vi "DO State Machine (array).vi"(0 "FPGA DO Loop Data in":T1={"DO"=[FALSE, FALSE, FALSE, FALSE, FALSE, FALSE, FALSE, FALSE, FALSE, FALSE, FALSE, FALSE, FALSE, FALSE, FALSE, FALSE, FALSE, FALSE, FALSE, FALSE, FALSE, FALSE, FALSE, FALSE, FALSE, FALSE, FALSE, FALSE, FALSE, FALSE, FALSE, FALSE], "Is Pulse"=[FALSE, FALSE, FALSE, FALSE, FALSE, FALSE, FALSE, FALSE, FALSE, FALSE, FALSE, FALSE, FALSE, FALSE, FALSE, FALSE, FALSE, FALSE, FALSE, FALSE, FALSE, FALSE, FALSE, FALSE, FALSE, FALSE, FALSE, FALSE, FALSE, FALSE, FALSE, FALSE], "Set Time uSec"=[0, 0, 0, 0, 0, 0, 0, 0, 0, 0, 0, 0, 0, 0, 0, 0, 0, 0, 0, 0, 0, 0, 0, 0, 0, 0, 0, 0, 0, 0, 0, 0], "Wait Time uSec"=[0, 0, 0, 0, 0, 0, 0, 0, 0, 0, 0, 0, 0, 0, 0, 0, 0, 0, 0, 0, 0, 0, 0, 0, 0, 0, 0, 0, 0, 0, 0, 0]}, 5 "#DO":u8, 7 "Value":bool, 9 "Time uSec":u32, 11 "Set":bool) -> (4 "FPGA DO Loop Data out":T1)   [LabVIEW 2019]
uses:
  TypeDef/FPGA DO Loop Data.ctl
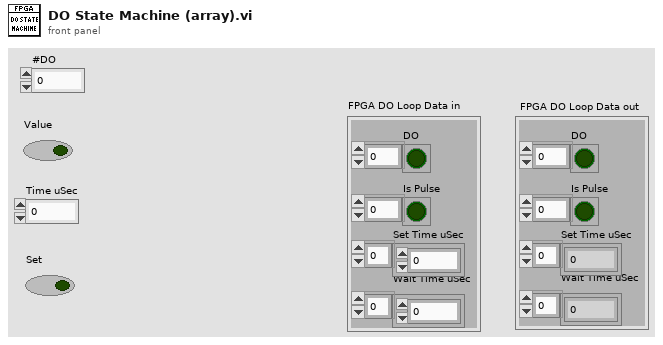
[diagram p1: front panel]
types:
  T1 = typedef "FPGA DO Loop Data.ctl" = cluster{"DO":bool[], "Is Pulse":bool[], "Set Time uSec":u32[], "Wait Time uSec":u32[]}
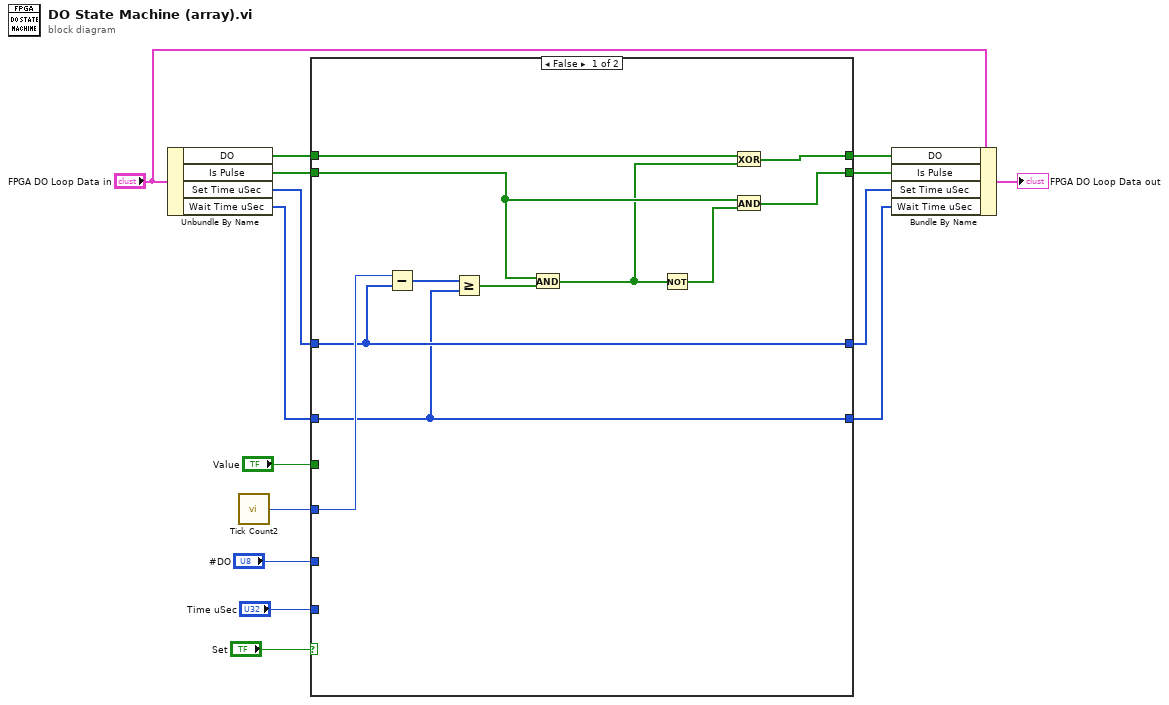
[diagram p0: block diagram]
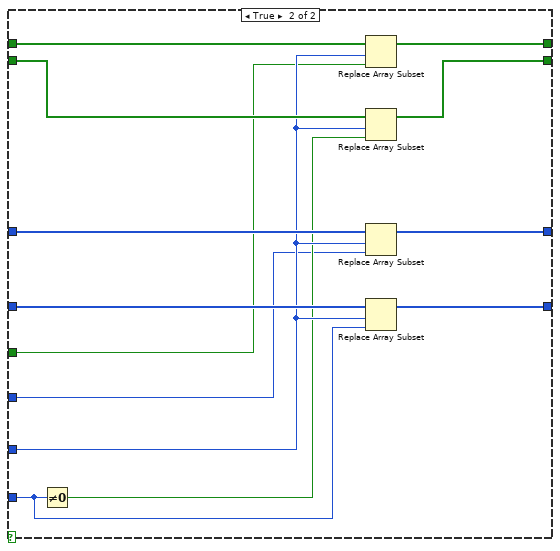
[diagram p2: hidden frame]
diagram:
  n1 = Unbundle By Name("FPGA DO Loop Data in") -> ("DO"=w11:bool[], "Is Pulse"=w3:bool[], "Set Time uSec"=w9:u32[], "Wait Time uSec"=w10:u32[])
  n2 = call "Tick Count2"() -> ("Tick Count(uSec)"=w12:u32)
  n3 = case shown="False" "Set" {
    tunnel: "Value" -> [_ w30]
    tunnel: [w20 w38] -> w7
    tunnel: w11 -> [w21 w39]
    tunnel: "Time uSec" -> [_ w27]
    tunnel: w12 -> [w26 w28]
    tunnel: [w24 w32] -> w5
    tunnel: w9 -> [w24 w35]
    tunnel: [w23 w33] -> w4
    tunnel: w10 -> [w23 w34]
    tunnel: [w16 w36] -> w2
    tunnel: w3 -> [w19 w37]
    tunnel: "#DO" -> [_ w31]
    frame False {
      n4 = Subtract(x=w26, y=w24) -> (x-y=w25:u32[])
      n5 = Greater Or Equal?(x=w25, y=w23) -> (x >= y?=w22:bool[])
      n6 = And(x=w19, y=w22) -> (x .and. y?=w18:bool[])
      n7 = Not(x=w18) -> (.not. x?=w17:bool[])
      n8 = Exclusive Or(1:w18, 2:w21) -> (0:w20:bool[])
      n9 = And(x=w19, y=w17) -> (x .and. y?=w16:bool[])
    }
    frame True {
      n10 = Not Equal To 0?(x=w27) -> (x != 0?=w29:bool)
      n11 = Replace Array Subset(array=w39, new element=w30, index=w31) -> (w38:bool[])
      n12 = Replace Array Subset(array=w37, new element=w29, index=w31) -> (w36:bool[])
      n13 = Replace Array Subset(array=w35, new element=w28, index=w31) -> (w32:u32[])
      n14 = Replace Array Subset(array=w34, new element=w27, index=w31) -> (w33:u32[])
    }
  }
  n15 = Bundle By Name(cluster="FPGA DO Loop Data in", "DO"=w7, "Is Pulse"=w2, "Set Time uSec"=w5, "Wait Time uSec"=w4) -> (→"FPGA DO Loop Data out":T1)
